vi "to.map.vi"(8 "error in":errorcluster, 11 "properties in":refnum<class "properties.lvclass">) -> (0 "error out":errorcluster, 2 "properties":map{string, string}(c390), 3 "properties out":refnum<class "properties.lvclass">)   [LabVIEW 2020, in "nominal types.lvlib" / "properties.lvclass"]
uses:
  properties.lvclass
  properties.lvclass/properties.ctl
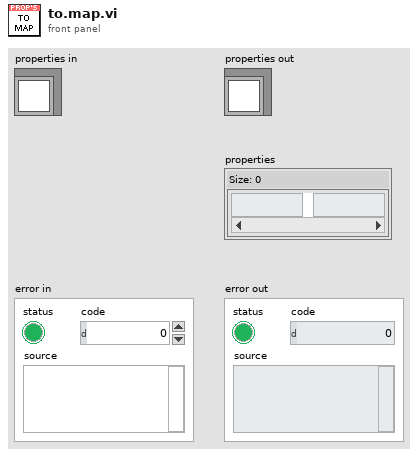
[diagram p1: front panel]
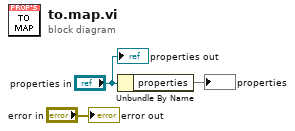
[diagram p0: block diagram]
diagram:
  n1 = Unbundle By Name("properties in") -> ("properties"=→"properties":map{string, string})
  "properties out" <- "properties in"
  "error out" <- "error in"
